vi "pump_Test.vi"() -> ()   [LabVIEW 2023, in "pump_Lib.lvlib"]
uses:
  pump_Lib.lvlib
  TypeDef/pair_Type.ctl
  TypeDef/pump_Type_Solo.ctl
  TypeDef/parametrs_Type.ctl
panel:
  in  "Параметры":T1
  out "Status":bool
  in  "Насос 2":T2={"Давление заданное"=0.3, "Давление MAX заданное"=100.0, "Давление в насосе"=0.0, "Давление в системе"=99.99, "Расход заданый"=0.0, "Расход текущий"=0.0, "Объём заданный"=0.0, "Объём текущий"=0.0, "Позиция насоса %"=0.0, "Ток двигателя"=0.0, "controlMsg"="", "Клапан k_sys"=FALSE, "Клапан k_res"=FALSE, "Клапан k_air"=FALSE, "Вверх"=FALSE, "Домой"=FALSE, "Вниз"=FALSE, "Старт расход"=FALSE, "Старт давление"=FALSE, "Сброс объёма"=FALSE, "Сброс давления Рсис"=FALSE, "Сброс давления Рнас"=FALSE, "Bits"={"plc_control"=FALSE, "lag_control"=FALSE, "mstop_control"=FALSE, "st_home"=FALSE, "error"=FALSE, "mstart"=FALSE, "pair"=FALSE, "startQ"=FALSE, "startP"=FALSE, "volume_Stop"=FALSE}} {"Ток двигателя" format="%#_5f"; "Расход текущий" format="%#_4f"; "Давление в системе" format="%.3f"; "Объём текущий" min=0.0 max=9999.0 step=0.0001 format="%#_4f"; "Объём заданный" min=0.0 max=9999.0 step=0.0001 format="%#_5f"; "Давление MAX заданное" min=0.0 max=100.0 step=0.01 format="%#_5f"; "Давление заданное" min=0.3 max=100.0 step=0.01 format="%#_5f"; "Расход заданый" min=-150.0 max=150.0 step=0.0001 format="%#_5f"; "Давление в насосе" format="%.3f"; "Позиция насоса %" scale=0.0..100.0 scale format="%.2f"}
  in  "Насос":T2={"Давление заданное"=0.3, "Давление MAX заданное"=100.0, "Давление в насосе"=0.0, "Давление в системе"=99.99, "Расход заданый"=0.0, "Расход текущий"=0.0, "Объём заданный"=0.0, "Объём текущий"=0.0, "Позиция насоса %"=0.0, "Ток двигателя"=0.0, "controlMsg"="", "Клапан k_sys"=FALSE, "Клапан k_res"=FALSE, "Клапан k_air"=FALSE, "Вверх"=FALSE, "Домой"=FALSE, "Вниз"=FALSE, "Старт расход"=FALSE, "Старт давление"=FALSE, "Сброс объёма"=FALSE, "Сброс давления Рсис"=FALSE, "Сброс давления Рнас"=FALSE, "Bits"={"plc_control"=FALSE, "lag_control"=FALSE, "mstop_control"=FALSE, "st_home"=FALSE, "error"=FALSE, "mstart"=FALSE, "pair"=FALSE, "startQ"=FALSE, "startP"=FALSE, "volume_Stop"=FALSE}} {"Ток двигателя" format="%#_5f"; "Расход текущий" format="%#_4f"; "Давление в системе" format="%.3f"; "Объём текущий" min=0.0 max=9999.0 step=0.0001 format="%#_4f"; "Объём заданный" min=0.0 max=9999.0 step=0.0001 format="%#_5f"; "Давление MAX заданное" min=0.0 max=100.0 step=0.01 format="%#_5f"; "Давление заданное" min=0.3 max=100.0 step=0.01 format="%#_5f"; "Расход заданый" min=-150.0 max=150.0 step=0.0001 format="%#_5f"; "Давление в насосе" format="%.3f"; "Позиция насоса %" scale=0.0..100.0 scale format="%.2f"}
  in  "Насосная система":T3={"Давление заданное"=0.3, "Давление в системе"=99.99, "Расход заданый"=0.0, "Расход текущий"=0.0, "Объём заданный"=0.0, "Объём текущий"=0.0, "Старт давление"=FALSE, "Старт расход"=FALSE, "Сброс объёма"=FALSE, "plc_control"=FALSE, "lag_control"=FALSE, "mstop_control"=FALSE, "Давление"={"АЦП CH 0"=0.0, "АЦП CH 1"=0.0, "АЦП CH 2"=0.0, "АЦП CH 3"=0.0, "АЦП CH 4"=0.0, "АЦП CH 5"=0.0, "АЦП CH 6"=0.0, "АЦП CH 7"=0.0}, "Modbus"={"Массив чтения"=[], "Массив записи"=[]}} {"Давление"."АЦП CH 7" format="%.3f"; "Давление"."АЦП CH 6" format="%.3f"; "Давление"."АЦП CH 5" format="%.3f"; "Давление"."АЦП CH 4" format="%.3f"; "Давление"."АЦП CH 3" format="%.3f"; "Давление"."АЦП CH 2" format="%.3f"; "Давление"."АЦП CH 1" format="%.3f"; "Давление"."АЦП CH 0" format="%.3f"; "Объём текущий" min=0.0 max=9999.0 step=0.0001 format="%#_4f"; "Объём заданный" min=0.0 max=9999.0 step=0.0001 format="%#_5f"; "Расход текущий" format="%#_4f"; "Расход заданый" min=-150.0 max=150.0 step=0.0001 format="%#_5f"; "Давление в системе" format="%.3f"; "Давление заданное" min=0.3 max=100.0 step=0.01 format="%#_5f"}
  in  "Stop":bool
  # "%"
  # "%"
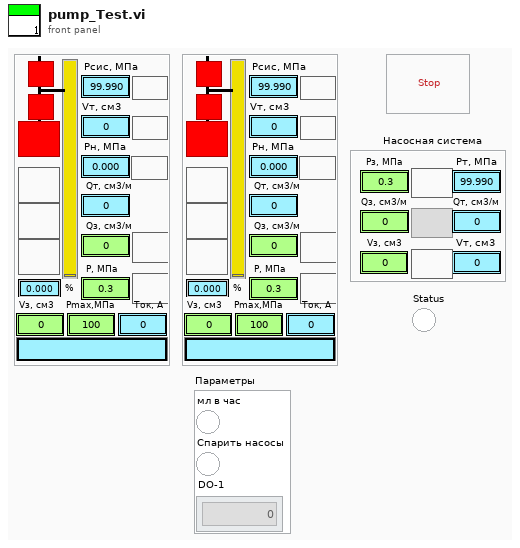
[diagram p1: front panel]
types:
  T1 = typedef "pump_Lib.lvlib/parametrs_Type.ctl" = cluster{"мл в час":bool, "Спарить насосы":bool, "DO-1":u16[]}
  T2 = typedef "pump_Lib.lvlib/pump_Type_Solo.ctl" = cluster{"Давление заданное":dbl, "Давление MAX заданное":dbl, "Давление в насосе":dbl, "Давление в системе":dbl, "Расход заданый":dbl, "Расход текущий":dbl, "Объём заданный":dbl, "Объём текущий":dbl, "Позиция насоса %":dbl, "Ток двигателя":dbl, "controlMsg":string, "Клапан k_sys":bool, "Клапан k_res":bool, "Клапан k_air":bool, "Вверх":bool, "Домой":bool, "Вниз":bool, "Старт расход":bool, "Старт давление":bool, "Сброс объёма":bool, "Сброс давления Рсис":bool, "Сброс давления Рнас":bool, "Bits":cluster{"plc_control":bool, "lag_control":bool, "mstop_control":bool, "st_home":bool, "error":bool, "mstart":bool, "pair":bool, "startQ":bool, "startP":bool, "volume_Stop":bool}}
  T3 = typedef "pump_Lib.lvlib/pair_Type.ctl" = cluster{"Давление заданное":dbl, "Давление в системе":dbl, "Расход заданый":dbl, "Расход текущий":dbl, "Объём заданный":dbl, "Объём текущий":dbl, "Старт давление":bool, "Старт расход":bool, "Сброс объёма":bool, "plc_control":bool, "lag_control":bool, "mstop_control":bool, "Давление":cluster{"АЦП CH 0":dbl, "АЦП CH 1":dbl, "АЦП CH 2":dbl, "АЦП CH 3":dbl, "АЦП CH 4":dbl, "АЦП CH 5":dbl, "АЦП CH 6":dbl, "АЦП CH 7":dbl}, "Modbus":cluster{"Массив чтения":u16[], "Массив записи":u16[]}}
  T4 = typedef "pump_Lib.lvlib/control_Type.ctl" = cluster{"IP Adress in":string, "control_Port_1 ref":refnum<vi>, "control_Port_2 ref":refnum<vi>, "control_Pair ref":refnum<vi>, "queue_Port 1":refnum<queue>, "queue_Port 2":refnum<queue>, "queue_Pair":refnum<queue>, "parametrs ref":refnum<vi>, "Stop Event":refnum<user-event>}
  T5 = typedef "pump_Lib.lvlib/pump_Type.ctl" = cluster{"Давление заданное":dbl, "Давление MAX заданное":dbl, "Давление в насосе":dbl, "Давление в системе":dbl, "Расход заданый":dbl, "Расход текущий":dbl, "Объём заданный":dbl, "Объём текущий":dbl, "Позиция насоса %":dbl, "Ток двигателя":dbl, "controlMsg":string, "Клапан k_sys":bool, "Клапан k_res":bool, "Клапан k_air":bool, "Вверх":bool, "Домой":bool, "Вниз":bool, "Старт расход":bool, "Старт давление":bool, "Сброс объёма":bool, "Сброс давления Рсис":bool, "Сброс давления Рнас":bool, "Bits":cluster{"plc_control":bool, "lag_control":bool, "mstop_control":bool, "st_home":bool, "error":bool, "mstart":bool, "pair":bool, "startQ":bool, "startP":bool, "volume_Stop":bool}}
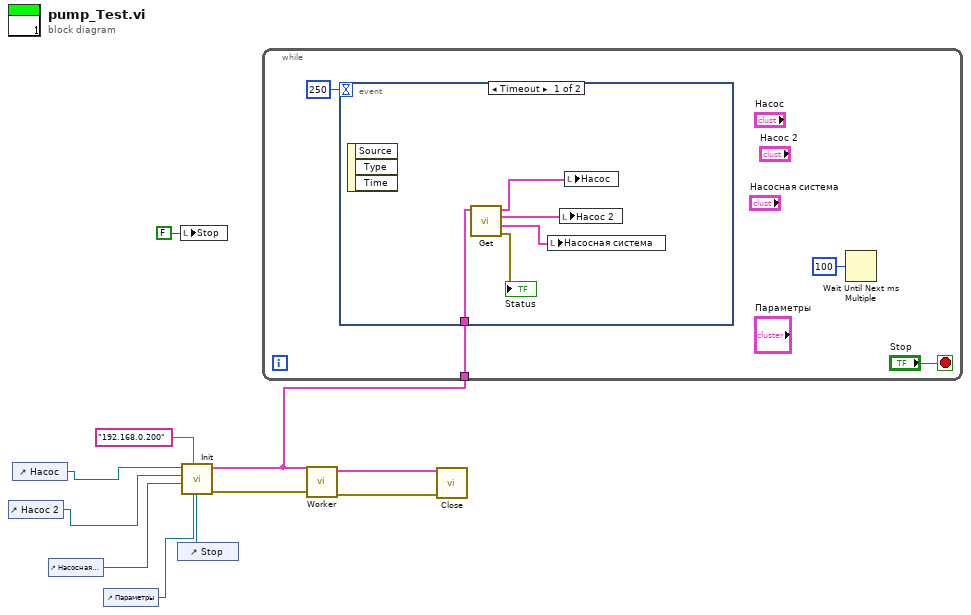
[diagram p0: block diagram]
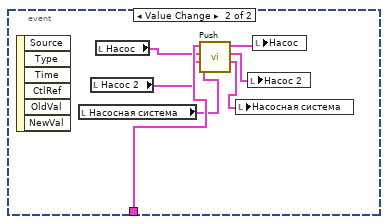
[diagram p2: hidden frame]
diagram:
  n1 = control-ref of="Насос 2"() -> (w2:refnum<vi>)
  n2 = control-ref of="Насос"() -> (w3:refnum<vi>)
  n3 = control-ref of="Насосная система"() -> (w6:refnum<vi>)
  n4 = control-ref of="Параметры"() -> (w1:refnum<vi>)
  n5 = control-ref of="Stop"() -> (w4:refnum<vi>)
  n6 = local write "Stop"(FALSE ("Stop")) -> ()
  n7 = call "Init.vi"("parametrs ref"=w1, "IP Adress in"="192.168.0.200", "Stop Event"=w4, "control_Pair ref"=w6, "control_Port_2 ref"=w2, "control_Port_1 ref"=w3) -> ("error out"=w11:errorcluster, "Управление ПЛК"=w8:T4)  [unwired: 4 in]
  n8 = while {
    tunnel: w8 -> [w12]
    stop <- "Stop" stop-if-true
    n9 = event shown="[0] Timeout" {
      selector: _ -> [_ _]
      dyn-events: _ -> [_ _]
      timeout: 250 -> [_ _]
      tunnel: w12 -> [w20 w27]
      event Timeout {
        n10 = event-data() -> ()  [unwired: 1 in, 3 out]
        n11 = call "Get.vi"("Управление ПЛК"=w20) -> ("error out"=→"Status":errorcluster, "Pair out"=w17:T3, "Port 2 out"=w18:T5, "Port 1 out"=w19:T5)  [unwired: 7 in]
        n12 = local write "Насосная система"(w17) -> ()
        n13 = local write "Насос 2"(w18) -> ()
        n14 = local write "Насос"(w19) -> ()
      }
      event Value Change {
        n15 = event-data() -> ()  [unwired: 1 in, 6 out]
        n16 = local read "Насосная система"() -> (w24:T3)
        n17 = local read "Насос 2"() -> (w25:T2)
        n18 = local read "Насос"() -> (w26:T2)
        n19 = call "Push.vi"("Pair in"=w24, "Port 2 in"=w25, "Port 1 in"=w26, "Управление ПЛК"=w27) -> ("Pair out"=w23:T3, "Port 2 out"=w22:T5, "Port 1 out"=w21:T5)  [unwired: 4 in, 1 out]
        n20 = local write "Насосная система"(w23) -> ()
        n21 = local write "Насос 2"(w22) -> ()
        n22 = local write "Насос"(w21) -> ()
      }
    }
    n23 = Wait Until Next ms Multiple(millisecond multiple=u32 100) -> ()  [unwired: 1 out]
  }
  n24 = call "Worker.vi"("Error In"=w11, "Управление ПЛК вход"=w8) -> ("Error Out"=w9:errorcluster, "Управление ПЛК выход"=w10:T4)  [unwired: 8 in]
  n25 = call "Close.vi"("Error In"=w9, "Управление ПЛК"=w10) -> ()  [unwired: 9 in, 1 out]
